vi "Keithley2100.vi"() -> ()   [LabVIEW 2020]
uses:
  SubVIs/Keithley2100_TypeDefinitions.llb/Button.ctl
  SubVIs/Keithley2100_TypeDefinitions.llb/Button_Rect.ctl
  <vilib>/Utility/miscctls.llb/LVPointTypeDef.ctl
  LabVIEW 2020 Toolkits/toolkits_lv2020_32bit/Synchronization.llb/SynchRefs_SetGet.ctl
  LabVIEW 2020 Toolkits/VI Server Toolkit/VI Server Libraries/VI Server_GetControl.llb/VI Server_STR_Get.vi
  LabVIEW 2020 Toolkits/VI Server Toolkit/VI Server Libraries/VI Server_GetControl.llb/VI Server_1D_Array_STR_Get.vi
  LabVIEW 2020 Toolkits/VI Server Toolkit/VI Server Libraries/VI Server_Set Controls.llb/Set STR Control.vi
  LabVIEW 2020 Toolkits/VI Server Toolkit/VI Server Toolkit LV2013.lvlib
panel:
  in  "DisableAutoUpdate":bool caption="Disable Auto Update"
  in  "DisableFP_Hide":bool caption="Disable FP Hide"
  out "System.Message":string caption="System Message"
  in  "Help":bool
  in  "FP.Hide":bool caption="FrontPanel.Hide"
  in  "EXIT":bool
  in  "Tab.Main":enum32{"DMM", "Sequence", "SETTINGS"}(tab)
  in  "Function.CONFIG":T1
  in  "Measurement.Range":string
  in  "Measure.Result":dbl format="%0.4f VDC"
  in  "Range.DOWN":bool
  in  "Range.UP":bool
  in  "Range.AUTO":bool
  in  "Function.Memory.LOCAL":T1
  in  "Function.SHIFT":T1
  in  "Function.Memory.RECALL":T1
  in  "Function.Memory.STORE":T1
  in  "Function.Trig.AUTO":bool
  in  "Function.Trig.SGL":T1
  in  "Function.NULL":T1
  in  "Function.Min/Max":T1
  in  "Function.%":T1
  in  "Function.Ratio":T1
  in  "Function.Digits":T1
  in  "Function.Filter":T1
  in  "Function.TEMP":bool
  in  "Function.CONT":bool
  in  "Function.FREQ":bool
  in  "Function.RESISTANCE":T2
  in  "Function.ACV":bool
  in  "Function.DCV":bool
  in  "TestCase.StepDescription":string caption="Step Description:"
  in  "TestCase.Execute.All":bool
  in  "TestCase.Execute.Selected":bool
  out "TestCase.SAVE.Success":bool
  in  "TestCase.SAVE":bool
  in  "SequenceFile.Open":bool
  in  "SequenceFile":path caption="Secuence File"
  in  "Settings.LOAD":bool
  in  "Settings.SAVE":bool
  in  "Settings.Number":i32=1 caption="Number" min=1 step=1
  in  "TestCase.Execute.Step.Pause":bool
  in  "TestCase.Execute.Steps":u16(ring) caption="Test Case: Pause Before Step" items=["1", "2"]
  in  "TestCase.Execute.ABORT":bool
  in  "TestCase.Execute.Next":bool
  in  "TestCase.Execute.Pause":bool
  out "TestCase.ExecutionTime":dbl caption="Execution Time:" format="%0.3f sec"
  in  "TestCase.Execution.StepTime":u32 caption="Seq. Execution: Step Time" format="%d msec"
  in  "TestCaseConfiguration":i32[](listbox) caption="Test Case Configuration"
  in  "DisableFP_OpenOnIDN_Call":bool caption="Disable FP Open\nON *IDN? Call"
  in  "Instr.Command2.Send":bool
  in  "Instr.Command2":string caption="Instrument: Command"
  in  "Instr.Command.Send":bool
  in  "Instr.Command":string caption="Instrument: Command"
  in  "UDP.Test.StringArray.Send":bool
  in  "UDP.TestStringsArray":string[](array[string]) caption="UDP: Test Strings Array"
  out "Instr.Responce":string caption="Instrument Responce"
  out "Instr.Command.Sent":string caption="Command: Sent"
  in  "VISA.ResourceName":refnum<visa-resource-name> caption="VISA Rresource Name"
  in  "Cont.Measurements.CycleTime":u32 caption="Continius Measurements:\nCycleTime"
  in  "UDP.Test.String2.Send":bool
  in  "UDP.Test.String2":string caption="UDP: Test String 2"
  in  "UDP.Port.BC":u16=58433 caption="UDP: Port.BC"
  in  "UDP.Port.RT":u16=58432 caption="UDP: Port.RT"
  in  "UDP.LocalPort.Write":u16=58434 caption="UDP: Local Port.Write"
  in  "UDP.IP.Address":string="234.5.6.7" caption="UDP: IP Address"
  in  "UDP.Test.String1.Send":bool
  in  "UDP.Test.String1":string caption="UDP: Test String 1"
  in  "UDP.Responce.String.Monitor":bool
  out "UDP.ExecEng.Message.String":string caption="UDP: Execution Engine Message String"
  out "error out":errorcluster={"status"=TRUE, "code"=1055, "source"="Property Node in VI Server Toolkit LV2013.lvlib:VI server_Set Control Value from String Format.vi:5200001->DMM6500_UDP_ExecEng_Instruction_APPLY.vi->DMM6500_UDP_MAIN.vi->Keithley2100.vi"}
  in  "error in":errorcluster
  # "DCI"
  # "ACI"
  # "PERIOD"
  # "4W"
  # "Mx+B"
  # "dBm"
  # "LIMITS"
  # "dB"
  # "M"
  # "Settings"
  # "Multicast IP addresses must be in the 224.0.0.0 to 239.255.255.255 range."
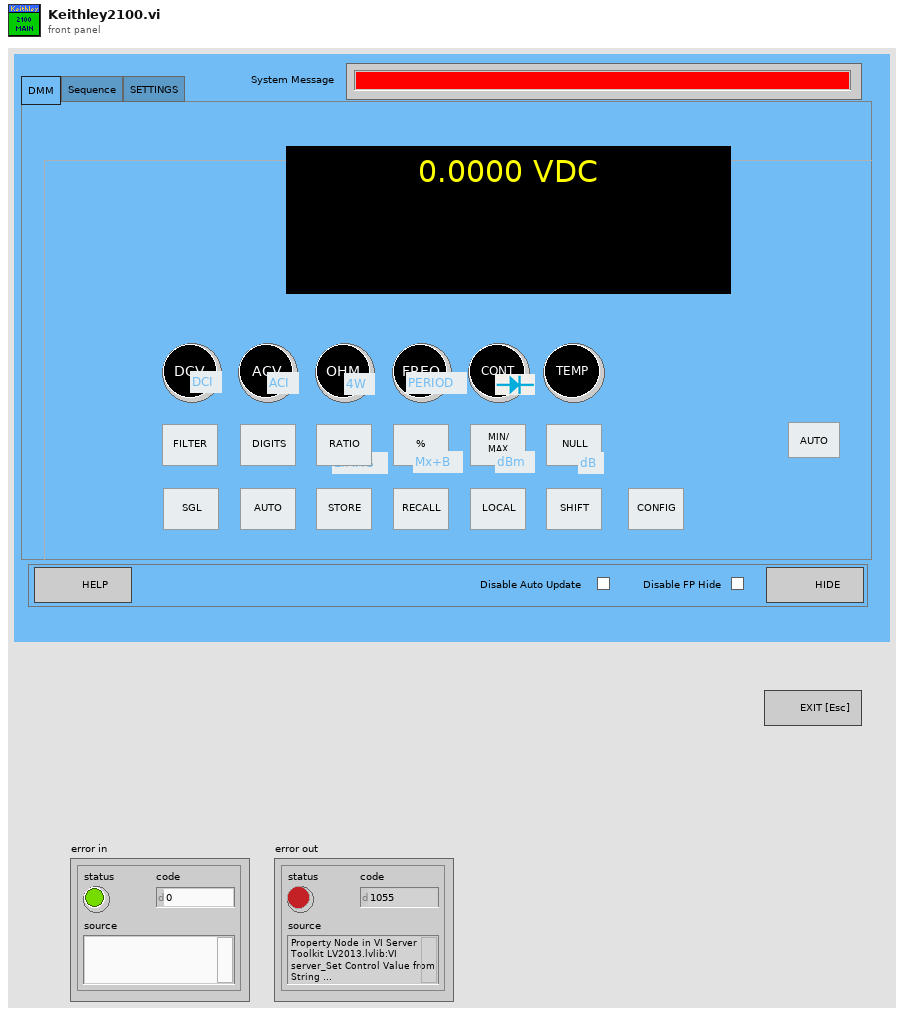
[diagram p1: front panel]
types:
  T1 = typedef "Button_Rect.ctl" = bool
  T2 = typedef "Button.ctl" = bool
  T3 = typedef "LVPointTypeDef.ctl" = cluster{"Horizontal":i16, "Vertical":i16}
  T4 = typedef "VI Server_RefsCluster.ctl" = cluster{"Labels":string[], "Refs":refnum<vi>[], "VI Ref":refnum<vi>}
  T5 = typedef "SynchRefs_SetGet.ctl" = enum16{"Set", "Get"}
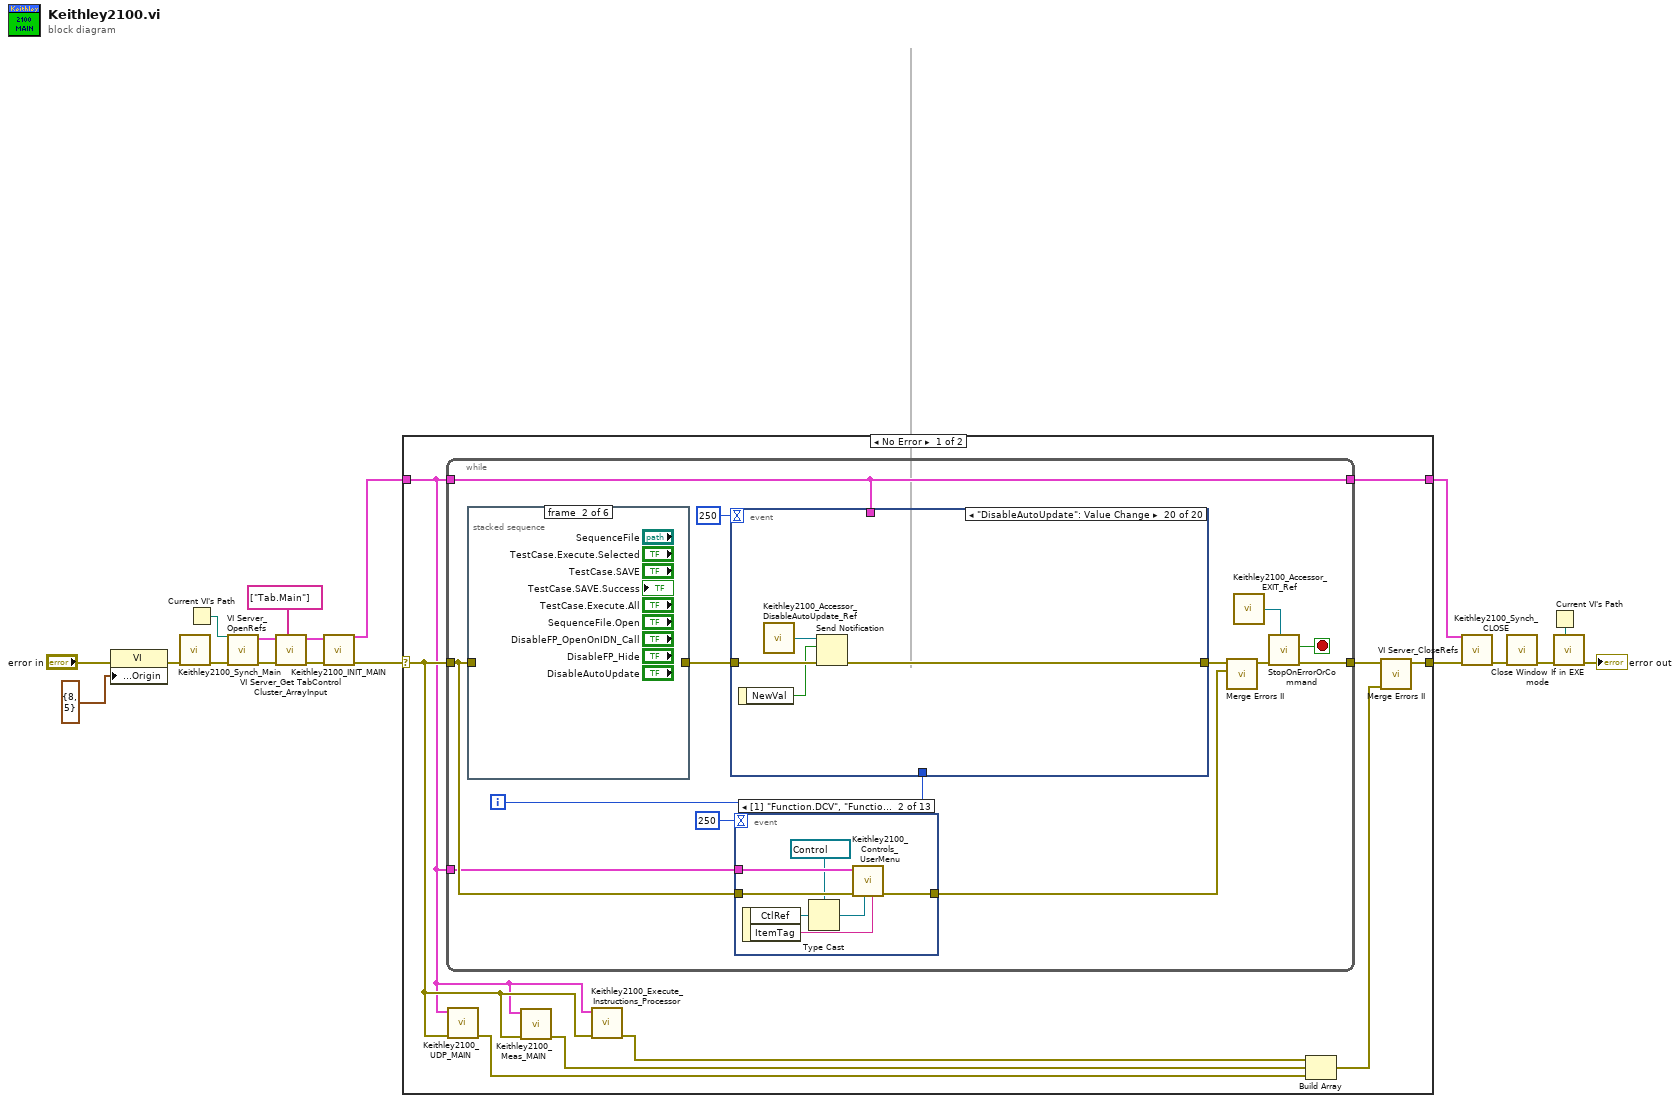
[diagram p0: block diagram]
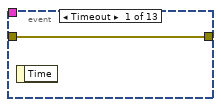
[diagram p2: hidden frame]
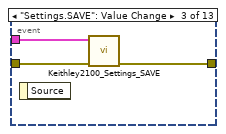
[diagram p3: hidden frame]
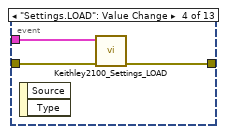
[diagram p4: hidden frame]
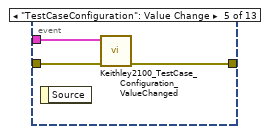
[diagram p5: hidden frame]
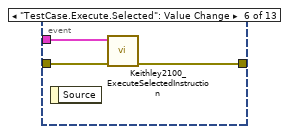
[diagram p6: hidden frame]
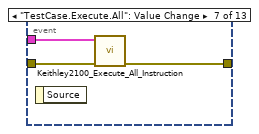
[diagram p7: hidden frame]
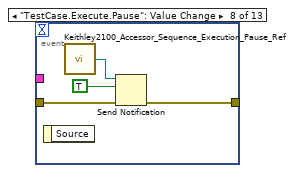
[diagram p8: hidden frame]
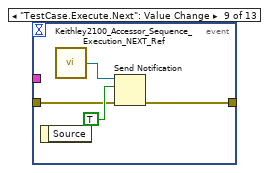
[diagram p9: hidden frame]
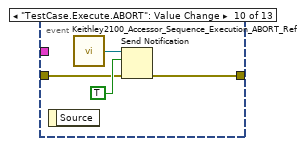
[diagram p10: hidden frame]
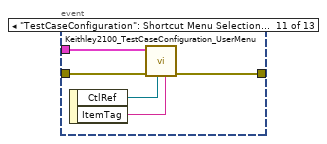
[diagram p11: hidden frame]
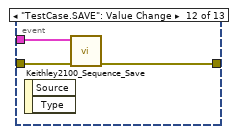
[diagram p12: hidden frame]
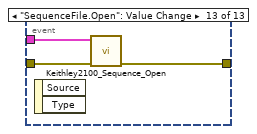
[diagram p13: hidden frame]
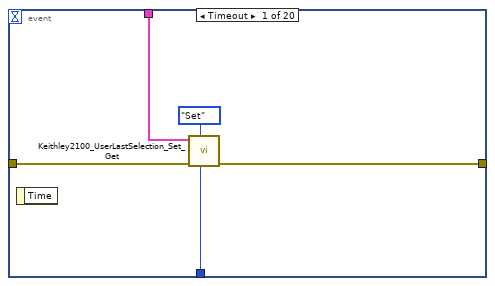
[diagram p14: hidden frame]
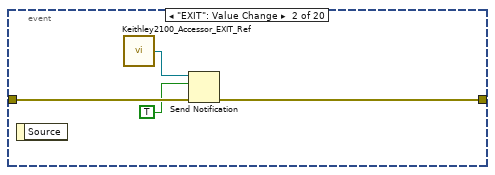
[diagram p15: hidden frame]
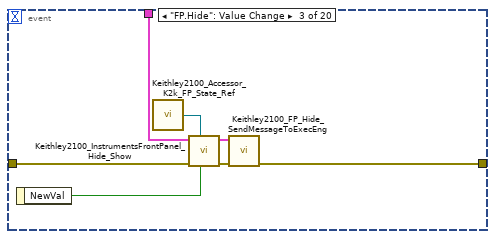
[diagram p16: hidden frame]
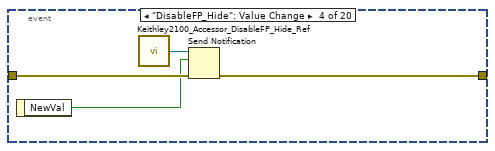
[diagram p17: hidden frame]
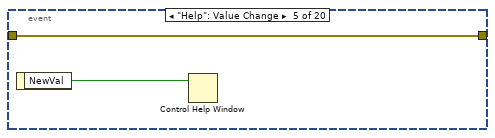
[diagram p18: hidden frame]
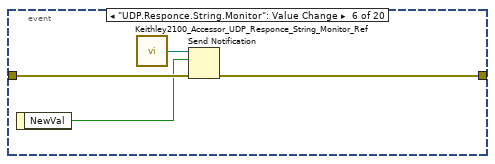
[diagram p19: hidden frame]
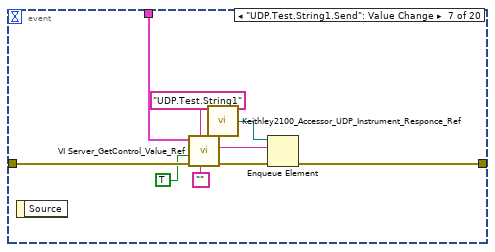
[diagram p20: hidden frame]
diagram:
  n1 = property class="VI"(error in="error in", "Front Panel Window:Origin"=T3 {"Horizontal"=8, "Vertical"=5}) -> (error out=w12:errorcluster)  [unwired: 1 in, 1 out]
  n2 = call "Keithley2100_Synch_Main.vi"("error in"=w12) -> ("error out"=w13:errorcluster)  [unwired: 10 in]
  n3 = Current VI's Path() -> (path=w17:path)
  n4 = call "VI Server_OpenRefs.vi"("error in"=w13, "VI Path"=w17) -> ("error out"=w14:errorcluster, "VI Server.RefsCluster"=w15:T4)  [unwired: 8 in]
  n5 = call "VI Server_Get TabControl Cluster_ArrayInput.vi"("TabControl Labels[]"=string[] ["Tab.Main"], "error in"=w14, "VI Server Cluster"=w15) -> ("error out"=w11:errorcluster, "VI Server Cluster.OUT"=w10:T4)  [unwired: 7 in]
  n6 = call "Keithley2100_INIT_MAIN.vi"("error in (no error)"=w11, "VI Server Cluster"=w10) -> ("error out"=w2:errorcluster, "VI Server Cluster DUP"=w9:T4)  [unwired: 8 in]
  n7 = case shown="No Error" w2 {
    selector: w2 -> [w21 w191]
    tunnel: [w25 w191] -> w1
    tunnel: w9 -> [w20 w190]
    tunnel: [w27 w190] -> w8
    frame No Error {
      n8 = while {
        tunnel: w21 -> [w31]
        tunnel: [w36] -> w22
        tunnel: w20 -> [w37]
        tunnel: [w37] -> w27
        tunnel: w20 -> [w29]
        i -> [w38]
        stop <- w35 stop-if-true
        n9 = stacked-sequence {
          tunnel: w31 -> [w189 _ _ _ _ _]
          tunnel: [w189 _ _ _ _ _] -> w40
          frame #0 {
          }
          frame #1 {
          }
          frame #2 {
          }
          frame #3 {
          }
          frame #4 {
          }
          frame #5 {
          }
        }
        n10 = event shown="[19] \"DisableAutoUpdate\": Value Change" {
          selector: _ -> [_ _ _ _ _ _ _ _ _ _ _ _ _ _ _ _ _ _ _ _]
          dyn-events: _ -> [_ _ _ _ _ _ _ _ _ _ _ _ _ _ _ _ _ _ _ _]
          timeout: 250 -> [_ _ _ _ _ _ _ _ _ _ _ _ _ _ _ _ _ _ _ _]
          tunnel: w40 -> [w90 w95 w101 w106 w108 w112 w121 w130 w138 w146 w157 w160 w163 w167 w168 w172 w177 w180 w184 w188]
          tunnel: w38 -> [w89 _ _ _ _ _ _ _ _ _ _ _ _ _ _ _ _ _ _ _]
          tunnel: [w88 w93 w102 w105 w108 w110 w119 w128 w132 w144 w154 w158 w161 w166 w169 w173 w176 w179 w182 w187] -> w33
          tunnel: w37 -> [w87 _ w98 _ _ _ w118 w127 w137 w143 _ w159 w162 _ w170 _ w175 w178 w183 _]
          event Timeout {
            n11 = event-data() -> ()  [unwired: 1 in, 1 out]
            n12 = call "Keithley2100_UserLastSelection_Set_Get.vi"("LoopCounter"=w89, "SynchRefs.Set/Get"=SynchRefs_SetGet."Set", "error in"=w90, "VI Server.RefsCluster"=w87) -> ("error out"=w88:errorcluster)  [unwired: 6 in, 1 out]
          }
          event "EXIT": Value Change {
            n13 = event-data() -> ()  [unwired: 1 in, 1 out]
            n14 = call "Keithley2100_Accessor_EXIT_Ref.vi"() -> ("EXIT"=w94:refnum<notifier>)  [unwired: 6 in]
            n15 = Send Notification(notification=TRUE, notifier=w94, error in (no error)=w95) -> (error out=w93:errorcluster)  [unwired: 1 out]
          }
          event "FP.Hide": Value Change {
            n16 = event-data() -> ("NewVal"=w97:bool)  [unwired: 1 in]
            n17 = call "Keithley2100_Accessor_K2k_FP_State_Ref.vi"() -> ("FP.State"=w96:refnum<notifier>)  [unwired: 6 in]
            n18 = call "Keithley2100_InstrumentsFrontPanel_Hide_Show.vi"("FP.Hide/Show"=w97, "FP.State"=w96, "error in (no error)"=w101, "VI Server Cluster"=w98) -> ("error out"=w100:errorcluster, "VI Server Cluster DUP"=w99:T4)  [unwired: 6 in]
            n19 = call "Keithley2100_FP_Hide_SendMessageToExecEng.vi"("error in (no error)"=w100, "VI Server Cluster"=w99) -> ("error out"=w102:errorcluster)  [unwired: 9 in]
          }
          event "DisableFP_Hide": Value Change {
            n20 = event-data() -> ("NewVal"=w103:bool)  [unwired: 1 in]
            n21 = call "Keithley2100_Accessor_DisableFP_Hide_Ref.vi"() -> ("DisableFP_Hide"=w104:refnum<notifier>)  [unwired: 6 in]
            n22 = Send Notification(notification=w103, notifier=w104, error in (no error)=w106) -> (error out=w105:errorcluster)  [unwired: 1 out]
          }
          event "Help": Value Change {
            n23 = event-data() -> ("NewVal"=w107:bool)  [unwired: 1 in]
            n24 = Control Help Window(1:w107) -> ()  [unwired: 1 in]
          }
          event "UDP.Responce.String.Monitor": Value Change {
            n25 = event-data() -> ("NewVal"=w109:bool)  [unwired: 1 in]
            n26 = call "Keithley2100_Accessor_UDP_Responce_String_Monitor_Ref.vi"() -> ("UDP.ExecEng.Command.String.Monitor"=w111:refnum<notifier>)  [unwired: 6 in]
            n27 = Send Notification(notification=w109, notifier=w111, error in (no error)=w112) -> (error out=w110:errorcluster)  [unwired: 1 out]
          }
          event "UDP.Test.String1.Send": Value Change {
            n28 = event-data() -> ()  [unwired: 1 in, 1 out]
            n29 = call-poly "VI Server_GetControl_Value_Ref.vi"("DataType"="", "Control.Label"="UDP.Test.String1", "error in"=w121, "SingleInstance"=TRUE, "VI Server.RefsCluster"=w118) -> ("error out"=w120:errorcluster, "Value"=w113:string)  [unwired: 3 in, 2 out]
            n30 = call "Keithley2100_Accessor_UDP_Instrument_Responce_Ref.vi"() -> ("UDP.Instrument.Responce.Q"=w114:refnum<queue>)  [unwired: 6 in]
            n31 = Enqueue Element(queue=w114, element=w113, error in (no error)=w120) -> (error out=w119:errorcluster)  [unwired: 1 in, 2 out]
          }
          event "UDP.Test.String2.Send": Value Change {
            n32 = event-data() -> ()  [unwired: 1 in, 1 out]
            n33 = call-poly "VI Server_GetControl_Value_Ref.vi"("DataType"="", "Control.Label"="UDP.Test.String2", "error in"=w130, "SingleInstance"=TRUE, "VI Server.RefsCluster"=w127) -> ("error out"=w129:errorcluster, "Value"=w122:string)  [unwired: 3 in, 2 out]
            n34 = call "Keithley2100_Accessor_UDP_Instrument_Responce_Ref.vi"() -> ("UDP.Instrument.Responce.Q"=w123:refnum<queue>)  [unwired: 6 in]
            n35 = Enqueue Element(queue=w123, element=w122, error in (no error)=w129) -> (error out=w128:errorcluster)  [unwired: 1 in, 2 out]
          }
          event "UDP.Test.StringArray.Send": Value Change {
            n36 = event-data() -> ()  [unwired: 1 in, 1 out]
            n37 = call-poly "VI Server_GetControl_Value_Ref.vi"("DataType"=string[] [], "Control.Label"="UDP.TestStringsArray", "error in"=w138, "SingleInstance"=TRUE, "VI Server.RefsCluster"=w137) -> ("error out"=w133:errorcluster, "Value"=w131:string[])  [unwired: 3 in, 2 out]
            n38 = for {
              tunnel: w133 -> [w141]
              tunnel: [w140] -> w132
              tunnel: w131 -> [w139] mode=indexing
              n39 = call "Keithley2100_Accessor_UDP_Instrument_Responce_Ref.vi"() -> ("UDP.Instrument.Responce.Q"=w142:refnum<queue>)  [unwired: 6 in]
              n40 = Enqueue Element(queue=w142, element=w139, error in (no error)=w141) -> (error out=w140:errorcluster)  [unwired: 1 in, 2 out]
            }
          }
          event "UDP.ExecEng.Message.String": Shortcut Menu Selection (User) {
            n41 = event-data() -> ("ItemTag"=w145:string)  [unwired: 1 in]
            n42 = case shown="\"Clear Indicator\"" w145 {
              tunnel: w146 -> [w147 w153]
              tunnel: [w147 w152] -> w144
              tunnel: w143 -> [_ w151]
              frame "", Default {
              }
              frame "Clear Indicator" {
                n43 = call-poly "VI Server_SetControl.vi"("New Value"="", "Label"="UDP.ExecEng.Message.String" ("Control.Label"), "error in"=w153, "Single Instance (T)"=TRUE ("SingleInstance"), "VI Server Cluster"=w151) -> ("error out"=w152:errorcluster)  [unwired: 4 in, 2 out]
              }
            }
          }
          event "VISA.ResourceName": Value Change {
            n44 = event-data() -> ("NewVal"=w155:refnum<visa-resource-name>)  [unwired: 1 in]
            n45 = call "Keithley2100_Accessor_VISA_Resource_Name_Ref.vi"() -> ("VISA resource name"=w156:refnum<notifier>)  [unwired: 6 in]
            n46 = Send Notification(notification=w155, notifier=w156, error in (no error)=w157) -> (error out=w154:errorcluster)  [unwired: 1 out]
          }
          event "Instr.Command.Send": Value Change {
            n47 = event-data() -> ()  [unwired: 1 in, 1 out]
            n48 = call "Keithley2100_WriteToInstrument.vi"("error in (no error)"=w160, "VI Server Cluster"=w159) -> ("error out"=w158:errorcluster)  [unwired: 9 in]
          }
          event "Instr.Command2.Send": Value Change {
            n49 = event-data() -> ()  [unwired: 1 in, 1 out]
            n50 = call "Keithley2100_WriteToInstrument2.vi"("error in (no error)"=w163, "VI Server Cluster"=w162) -> ("error out"=w161:errorcluster)  [unwired: 9 in]
          }
          event "Cont.Measurements.CycleTime": Value Change {
            n51 = event-data() -> ("NewVal"=w164:u32)  [unwired: 1 in]
            n52 = call "Keithley2100_Accessor_Cont_Measurements_CycleTime_Ref.vi"() -> ("Cont.Measurements.CycleTime"=w165:refnum<notifier>)  [unwired: 6 in]
            n53 = Send Notification(notification=w164, notifier=w165, error in (no error)=w167) -> (error out=w166:errorcluster)  [unwired: 1 out]
          }
          event Value Change {
            n54 = event-data() -> ()  [unwired: 1 in, 1 out]
            n55 = call "Keithley2100_Trigger_SGL.vi"("error in (no error)"=w168, "VI Server.RefsCluster"=w170) -> ("error out"=w169:errorcluster)  [unwired: 9 in]
          }
          event "Function.Trig.AUTO": Value Change {
            n56 = event-data() -> ("NewVal"=w171:bool)  [unwired: 1 in]
            n57 = call "Keithley2100_Trigger_AUTO.vi"("Trigger.AUTO"=w171, "error in (no error)"=w172) -> ("error out"=w173:errorcluster)  [unwired: 9 in]
          }
          event "Function.DCV", "Function.ACV", "Function.FREQ", "Function.CONT", "Function.TEMP": Value Change {
            n58 = event-data() -> ("CtlRef"=w174:refnum<vi>)  [unwired: 1 in]
            n59 = call "Keithley2100_MeasurementCommand_Send.vi"("CtlRef"=w174, "error in (no error)"=w177, "VI Server Cluster"=w175) -> ("error out"=w176:errorcluster)  [unwired: 8 in]
          }
          event "Range.AUTO": Value Change {
            n60 = event-data() -> ()  [unwired: 1 in, 1 out]
            n61 = call "Keithley2100_Measurement_Range_AUTO.vi"("error in (no error)"=w180, "VI Server Cluster"=w178) -> ("error out"=w179:errorcluster)  [unwired: 9 in]
          }
          event "Range.UP", "Range.DOWN": Value Change {
            n62 = event-data() -> ("CtlRef"=w181:refnum<vi>)  [unwired: 1 in]
            n63 = call "Keithley2100_Range_Up_Down_Set.vi"("CtlRef"=w181, "error in (no error)"=w184, "VI Server.RefsCluster"=w183) -> ("error out"=w182:errorcluster)  [unwired: 8 in]
          }
          event "DisableAutoUpdate": Value Change {
            n64 = event-data() -> ("NewVal"=w186:bool)  [unwired: 1 in]
            n65 = call "Keithley2100_Accessor_DisableAutoUpdate_Ref.vi"() -> ("DisableAutoUpdate"=w185:refnum<notifier>)  [unwired: 6 in]
            n66 = Send Notification(notification=w186, notifier=w185, error in (no error)=w188) -> (error out=w187:errorcluster)  [unwired: 1 out]
          }
        }
        n67 = event shown="[1] \"Function.DCV\", \"Function.ACV\", \"Function.RESISTANCE\", \"Function.FREQ\", \"Function.CONT\", \"Function.TEMP\", \"Function.Filter\", \"Function.Digits\", \"Function.Ratio\", \"Function.%\", \"Function.Min/Max\", \"Function.NULL\", \"Function.Trig.SGL\", \"Function.Trig.AUTO\", \"Function.Memory.STORE\", \"Function.Memory.RECALL\", \"Function.SHIFT\", \"Function.Memory.LOCAL\", \"Function.CONFIG\": Shortcut Menu Selection (User)" {
          selector: _ -> [_ _ _ _ _ _ _ _ _ _ _ _ _]
          dyn-events: _ -> [_ _ _ _ _ _ _ _ _ _ _ _ _]
          timeout: 250 -> [_ _ _ _ _ _ _ _ _ _ _ _ _]
          tunnel: w31 -> [w41 w47 w51 w54 w57 w60 w63 w67 w70 w74 w80 w83 w86]
          tunnel: [w41 w46 w49 w53 w55 w58 w61 w66 w69 w73 w79 w81 w84] -> w30
          tunnel: w29 -> [_ w48 w50 w52 w56 w59 w62 _ _ _ w76 w82 w85]
          event Timeout {
            n68 = event-data() -> ()  [unwired: 1 in, 1 out]
          }
          event "Function.DCV", "Function.ACV", "Function.FREQ", "Function.CONT", "Function.TEMP", "Function.Trig.AUTO": Shortcut Menu Selection (User) {
            n69 = event-data() -> ("CtlRef"=w45:refnum<vi>, "ItemTag"=w42:string)  [unwired: 1 in]
            n70 = Type Cast(type=refnum<vi> refnum ("Control Ref"), x=w45) -> (*(type *) &x=w44:refnum<vi>)
            n71 = call "Keithley2100_Controls_UserMenu.vi"("ItemTag"=w42, "Control Ref"=w44, "error in (no error)"=w47, "VI Server Cluster"=w48) -> ("error out"=w46:errorcluster)  [unwired: 7 in]
          }
          event "Settings.SAVE": Value Change {
            n72 = event-data() -> ()  [unwired: 1 in, 1 out]
            n73 = call "Keithley2100_Settings_SAVE.vi"("error in (no error)"=w51, "VI Server Cluster"=w50) -> ("error out"=w49:errorcluster)  [unwired: 9 in]
          }
          event "Settings.LOAD": Value Change {
            n74 = event-data() -> ()  [unwired: 1 in, 2 out]
            n75 = call "Keithley2100_Settings_LOAD.vi"("error in (no error)"=w54, "VI Server Cluster"=w52) -> ("error out"=w53:errorcluster)  [unwired: 9 in]
          }
          event "TestCaseConfiguration": Value Change {
            n76 = event-data() -> ()  [unwired: 1 in, 1 out]
            n77 = call "Keithley2100_TestCase_Configuration_ValueChanged.vi"("error in"=w57, "VI Server.RefsCluster"=w56) -> ("error out"=w55:errorcluster)  [unwired: 8 in, 1 out]
          }
          event "TestCase.Execute.Selected": Value Change {
            n78 = event-data() -> ()  [unwired: 1 in, 1 out]
            n79 = call "Keithley2100_ExecuteSelectedInstruction.vi"("error in (no error)"=w60, "VI Server Cluster"=w59) -> ("error out"=w58:errorcluster)  [unwired: 9 in]
          }
          event "TestCase.Execute.All": Value Change {
            n80 = event-data() -> ()  [unwired: 1 in, 1 out]
            n81 = call "Keithley2100_Execute_All_Instruction.vi"("error in (no error)"=w63, "VI Server Cluster"=w62) -> ("error out"=w61:errorcluster)  [unwired: 9 in]
          }
          event "TestCase.Execute.Pause": Value Change {
            n82 = event-data() -> ()  [unwired: 1 in, 1 out]
            n83 = call "Keithley2100_Accessor_Sequence_Execution_Pause_Ref.vi"() -> ("SequenceExecution.PAUSE"=w64:refnum<notifier>)  [unwired: 6 in]
            n84 = Send Notification(notification=TRUE, notifier=w64, error in (no error)=w67) -> (error out=w66:errorcluster)  [unwired: 1 out]
          }
          event "TestCase.Execute.Next": Value Change {
            n85 = event-data() -> ()  [unwired: 1 in, 1 out]
            n86 = call "Keithley2100_Accessor_Sequence_Execution_NEXT_Ref.vi"() -> ("SequenceExecution.NEXT"=w68:refnum<notifier>)  [unwired: 6 in]
            n87 = Send Notification(notification=TRUE, notifier=w68, error in (no error)=w70) -> (error out=w69:errorcluster)  [unwired: 1 out]
          }
          event "TestCase.Execute.ABORT": Value Change {
            n88 = event-data() -> ()  [unwired: 1 in, 1 out]
            n89 = call "Keithley2100_Accessor_Sequence_Execution_ABORT_Ref.vi"() -> ("SequenceExecution.ABORT"=w72:refnum<notifier>)  [unwired: 6 in]
            n90 = Send Notification(notification=TRUE, notifier=w72, error in (no error)=w74) -> (error out=w73:errorcluster)  [unwired: 1 out]
          }
          event "TestCaseConfiguration": Shortcut Menu Selection (User) {
            n91 = event-data() -> ("CtlRef"=w78:refnum<vi>, "ItemTag"=w77:string)  [unwired: 1 in]
            n92 = call "Keithley2100_TestCaseConfiguration_UserMenu.vi"("ItemTag"=w77, "MulticolumnListbox in"=w78, "error in (no error)"=w80, "VI Server Cluster"=w76) -> ("error out"=w79:errorcluster)  [unwired: 7 in]
          }
          event "TestCase.SAVE": Value Change {
            n93 = event-data() -> ()  [unwired: 1 in, 2 out]
            n94 = call "Keithley2100_Sequence_Save.vi"("error in (no error)"=w83, "VI Server Cluster"=w82) -> ("error out"=w81:errorcluster)  [unwired: 9 in]
          }
          event "SequenceFile.Open": Value Change {
            n95 = event-data() -> ()  [unwired: 1 in, 2 out]
            n96 = call "Keithley2100_Sequence_Open.vi"("error in (no error)"=w86, "VI Server Cluster"=w85) -> ("error out"=w84:errorcluster)  [unwired: 9 in]
          }
        }
        n97 = call "Merge Errors II.vi"("error in 2 (no error)"=w30, "error in 1 (no error)"=w33) -> ("error out.DUP"=w32:errorcluster)  [unwired: 4 in, 1 out]
        n98 = call "Keithley2100_Accessor_EXIT_Ref.vi"() -> ("EXIT"=w34:refnum<notifier>)  [unwired: 6 in]
        n99 = call "StopOnErrorOrCommand.vi"("STOP"=w34, "error in (no error)"=w32) -> ("error out"=w36:errorcluster, "STOP"=w35:bool)  [unwired: 8 in]
      }
      n100 = call "Keithley2100_UDP_MAIN.vi"("error in (no error)"=w21, "VI Server.RefsCluster"=w20) -> ("error out"=w26:errorcluster)  [unwired: 9 in]
      n101 = call "Keithley2100_Meas_MAIN.vi"("error in (no error)"=w21, "VI Server.RefsCluster"=w20) -> ("error out"=w23:errorcluster)  [unwired: 9 in]
      n102 = call "Keithley2100_Execute_Instructions_Processor.vi"("error in (no error)"=w21, "VI Server.RefsCluster"=w20) -> ("error out"=w19:errorcluster)  [unwired: 9 in]
      n103 = Build Array(w19, w23, w26) -> (w24:errorcluster[])
      n104 = call "Merge Errors II.vi"("error array in"=w24, "error in 1 (no error)"=w22) -> ("error out.DUP"=w25:errorcluster)  [unwired: 4 in, 1 out]
    }
    frame Error {
    }
  }
  n105 = call "VI Server_CloseRefs.vi"("error in"=w1, "VI Server.RefsCluster"=w8) -> ("error out"=w7:errorcluster)  [unwired: 9 in]
  n106 = call "Keithley2100_Synch_CLOSE.vi"("error in"=w7) -> ("error out"=w5:errorcluster)  [unwired: 10 in]
  n107 = Current VI's Path() -> (path=w3:path)
  n108 = call "Close Window If in EXE mode.vi"("TopLevelVI Path"=w3, "error in"=w5) -> ("error out"=→"error out":errorcluster)  [unwired: 9 in]
